vi "Required Font-Scale.vi"   [LabVIEW 2020, in "image.lvlib"]
doc: "Compute the size of text for the given parameters."
uses:
  image.lvlib
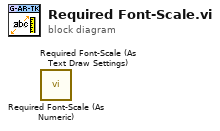
[diagram p0: block diagram]
diagram:
  n1 = call "Required Font-Scale (As Numeric).vi"() -> ()  [unwired: 10 in, 2 out]
  n2 = call "Required Font-Scale (As Text Draw Settings).vi"() -> ()  [unwired: 10 in, 2 out]
